vi "循环的数据输入输出.vi"() -> ()   [LabVIEW 2010]
panel:
  out "波形图表2":dbl(graph)
  out "波形图表":dbl(graph)
  in  "滑动杆2":dbl(slide) scale=0.0..10.0
  in  "滑动杆":dbl(slide) scale=0.0..10.0
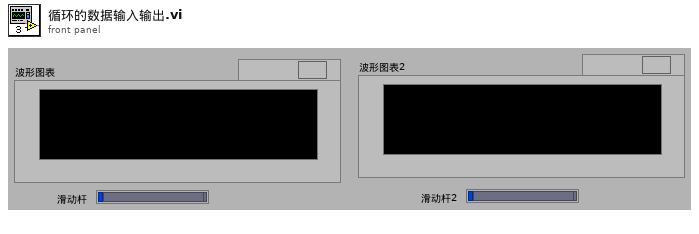
[diagram p1: front panel]
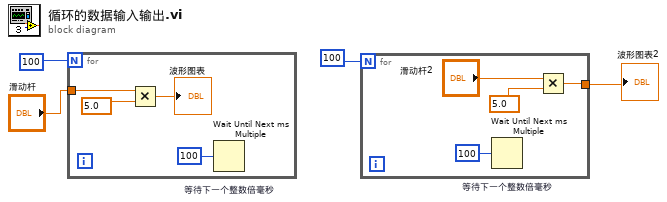
[diagram p0: block diagram]
diagram:
  n1 = for {
    N: 100 -> [_]
    tunnel: "滑动杆" -> [w8]
    n2 = Multiply(x=w8, y=5.0) -> (x*y=→"波形图表":dbl)
    n3 = Wait Until Next ms Multiple "等待下一个整数倍毫秒"(millisecond multiple=u32 100) -> ()  [unwired: 1 out]
  }
  n4 = for {
    N: 100 -> [_]
    tunnel: [w10] -> w1
    n5 = Wait Until Next ms Multiple "等待下一个整数倍毫秒"(millisecond multiple=u32 100) -> ()  [unwired: 1 out]
    n6 = Multiply(x="滑动杆2", y=5.0) -> (x*y=w10:dbl)
  }
  "波形图表2" <- w1
